vi "MessageQueue_ReleaseQueue.vi"(0 "QueueIn":refnum<queue>, 5 "ErrorIn":errorcluster) -> (15 "Name":string, 17 "RemainingElements":T1[](array[typedef]), 19 "ErrorOut":errorcluster)   [LabVIEW 2016]
doc: "Gibt einen Message Queue frei\n\nsige / 4.12.13"
uses:
  private/MessageQueue.MessageTypeDef.ctl
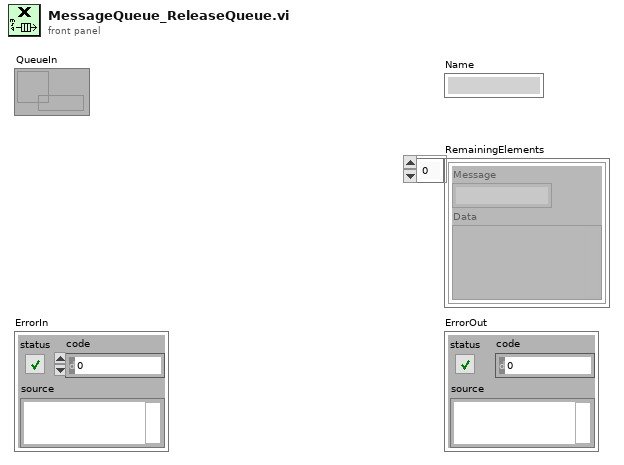
[diagram p1: front panel]
types:
  T1 = typedef "MessageQueue.MessageTypeDef.ctl" = cluster{"Message":string, "Data":variant}
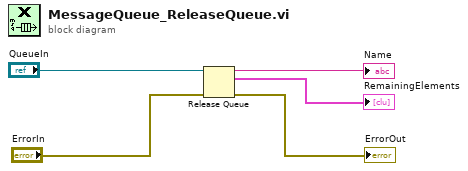
[diagram p0: block diagram]
diagram:
  n1 = Release Queue(queue="QueueIn", error in (no error)="ErrorIn") -> (queue name=→"Name":string, remaining elements=→"RemainingElements":T1[], error out=→"ErrorOut":errorcluster)  [unwired: 1 in]
